vi "Add PCC.vi"(6 "DeviceID":T1, 8 "error in":errorcluster, 11 "Startup Optimization in":refnum<class "Startup Optimization.lvclass">) -> (0 "error out":errorcluster, 3 "Startup Optimization out":refnum<class "Startup Optimization.lvclass">)   [LabVIEW 2018, in "Startup Optimization Actor.lvlib" / "Startup Optimization.lvclass"]
uses:
  Startup Optimization.lvclass
  <vilib>/ORNL/CSEISMIC DDS/CSEISMIC DDS Base/Data Types/Controls/DeviceID.ctl
  Startup Optimization.lvclass/Startup Optimization.ctl
  <vilib>/ORNL/CSEISMIC DDS/CSEISMIC DDS Base/CSEISMIC DDS.lvclass
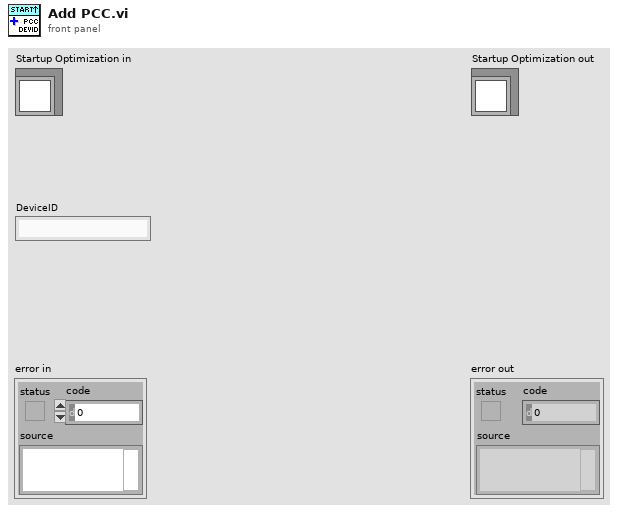
[diagram p1: front panel]
types:
  T1 = typedef "CSEISMIC DDS.lvlib/CSEISMIC DDS.lvclass/DeviceID.ctl" = string
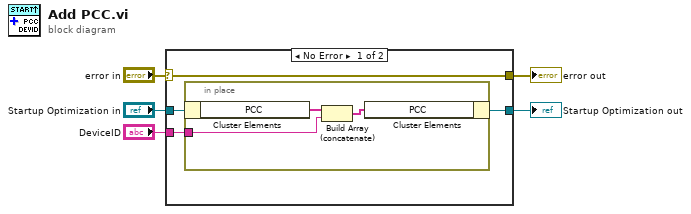
[diagram p0: block diagram]
diagram:
  n1 = case shown="No Error" "error in" {
    selector: "error in" -> [w9 w13]
    tunnel: [w9 w13] -> w4
    tunnel: [w6 w14] -> w2
    tunnel: "Startup Optimization in" -> [w7 w14]
    tunnel: "DeviceID" -> [w8 _]
    frame No Error {
      n2 = in-place {
        in-place-border: w8 -> [w12]
        n3 = in-place-cluster #1(w7) -> ("PCC"=w11:T1[])
        n4 = Build Array (concatenate)(w11, w12) -> (w10:T1[])
        n5 = in-place-cluster #1("PCC"=w10) -> (w6:refnum<class "Startup Optimization.lvclass">)
      }
    }
    frame Error {
    }
  }
  "error out" <- w4
  "Startup Optimization out" <- w2
